vi "Convert TimeString To TimeStamp(YYYY_MM_DD).vi"(1 "时间字符串（H:MM）":string="2016-01-18") -> (0 "date time rec":T1)   [LabVIEW 2015]
uses:
  <vilib>/Utility/miscctls.llb/LVDateTimeRec.ctl
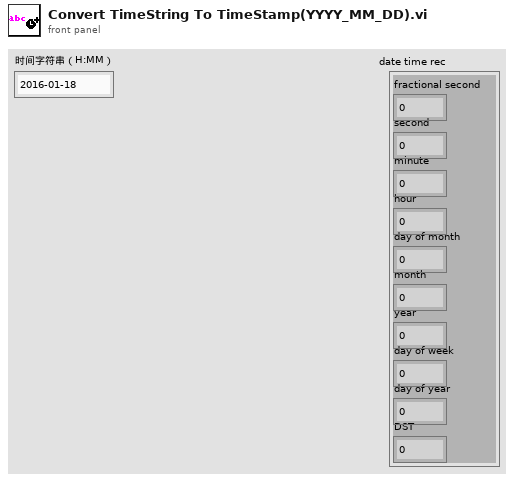
[diagram p1: front panel]
types:
  T1 = typedef "LVDateTimeRec.ctl" = cluster{"fractional second":dbl, "second":i32, "minute":i32, "hour":i32, "day of month":i32, "month":i32, "year":i32, "day of week":i32, "day of year":i32, "DST":i32}
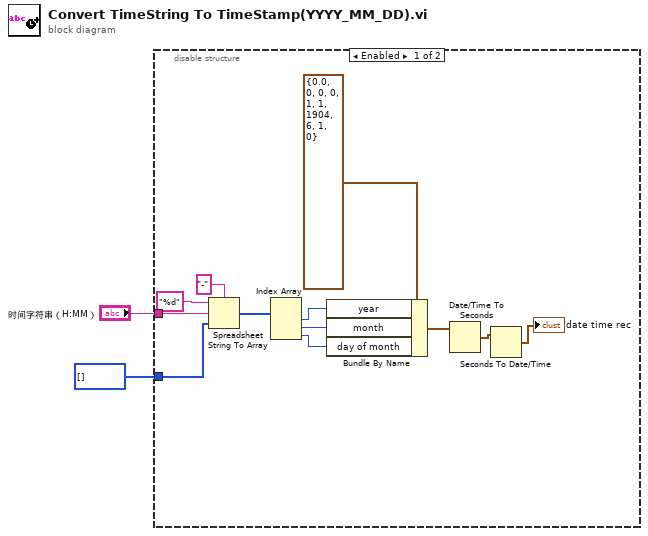
[diagram p0: block diagram]
diagram:
  n1 = disable-structure shown="Enabled" {
    disable-tunnel: "时间字符串（H:MM）" -> [w12 _]
    disable-tunnel: i32[] [] -> [w13 _]
    frame Enabled {
      n2 = Spreadsheet String To Array(delimiter (Tab)="-", format string="%d", spreadsheet string=w12, array type (2D Dbl)=w13) -> (array=w9:i32[])
      n3 = Index Array(array=w9) -> (element #1=w8:i32, element #2=w7:i32, element #3=w6:i32)  [unwired: 3 in]
      n4 = Bundle By Name(cluster=T1 {"fractional second"=0.0, "second"=0, "minute"=0, "hour"=0, "day of month"=1, "month"=1, "year"=1904, "day of week"=6, "day of year"=1, "DST"=0} ("date time rec"), "year"=w8, "month"=w7, "day of month"=w6) -> (w5:T1)
      n5 = Date/Time To Seconds(2:w5) -> (0:w4:timestamp)  [unwired: 1 in]
      n6 = Seconds To Date/Time(time stamp (now)=w4) -> (date time rec=→"date time rec":T1)  [unwired: 1 in]
    }
    frame Disabled {
    }
  }
